vi "Arm AV Measurement.vi"(0 "VISA resource name":refnum<visa-resource-name>, 11 "error in (no error)":errorcluster) -> (4 "VISA resource name out":refnum<visa-resource-name>, 15 "error out":errorcluster)   [LabVIEW 2020, in "Keithley 648X Series.lvlib"]
doc: "Arms the AV (Alternating Voltage) ohms mode. The instrument will start taking AV readings the next time it is initiated. This VI must be used prior (recommended immediately prior) to the <b>Read AV Measurement</b> VI.\n\n<b>Notes:</b>\n1) The data buffer cannot contain normal readings and the current autorange cannot be enabled when this VI is used.\n2) This VI is only valid for Keithley 6487."
uses:
  <instrlib>/Keithley 648X Series/Keithley 648X Series.lvlib
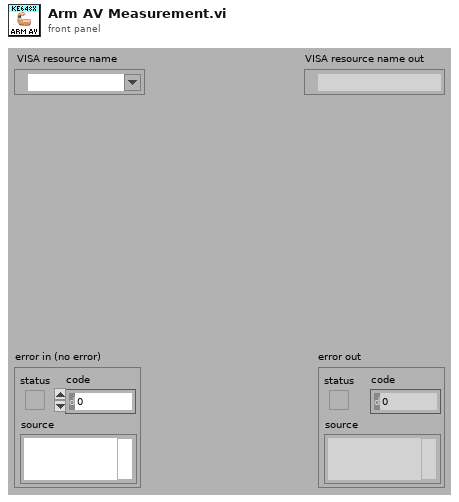
[diagram p1: front panel]
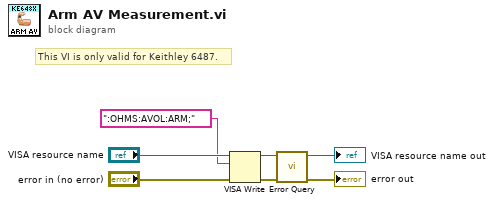
[diagram p0: block diagram]
diagram:
  # "This VI is only valid for Keithley 6487."
  n1 = VISA Write(VISA resource name="VISA resource name", write buffer=":OHMS:AVOL:ARM;", error in (no error)="error in (no error)") -> (VISA resource name out=w3:refnum<visa-resource-name>, error out=w2:errorcluster)  [unwired: 1 out]
  n2 = call <instrlib>:"Error Query.vi"("error in (no error)"=w2, "VISA resource name"=w3) -> ("error out"=→"error out":errorcluster, "VISA resource name out"=→"VISA resource name out":refnum<visa-resource-name>)  [unwired: 6 in, 2 out]
